vi "GetCalibration.vi"(1 "Handle":i32, 2 "Axis":u32) -> (0 "Calibration (um)":dbl format="%.3f")   [LabVIEW 2012]
uses:
  Madlib.dll
panel:
  # "This VI is a simple example of how to\nget the calibration on a particular axis\nof your nanopositioner."
  # "X = 1\nY = 2\nZ = 3"
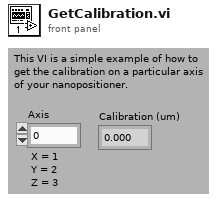
[diagram p1: front panel]
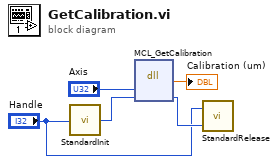
[diagram p0: block diagram]
diagram:
  n1 = call "StandardInit.vi"("Incoming Handle"="Handle") -> ("Outgoing Handle"=w3:i32)
  n2 = dll-call lib="C:/Users/Labview/Desktop/SRR/Madlib_x64/Labview Examples/MADLib.dll" fn="MCL_GetCalibration"("axis"="Axis", "handle"=w3) -> (→"Calibration (um)":dbl, "handle"=w2:i32)  [unwired: 4 in, 2 out]
  n3 = call "StandardRelease.vi"("Outgoing Handle"=w2, "Incoming Handle"="Handle") -> ()  [unwired: 1 in]
